vi "EmergencyStopAll.vi"() -> ()   [LabVIEW 2010]
uses:
  GenericDriveCommand.ctl
  DriveConfigGlobal.vi
panel:
  in  "stop":bool
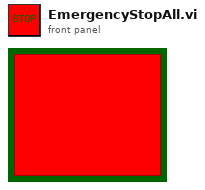
[diagram p1: front panel]
types:
  T1 = typedef "GenericDriveCommand.ctl" = string
  T2 = typedef "AxisConfigCluster.ctl" = cluster{"Channel Properties":T3, "Static Drive Configuration":T4}
  T3 = typedef "DriveProperties.ctl" = cluster{"Channel Name":string, "Vel. Default":dbl, "Acc. Default":dbl, "Vel. Max":dbl, "Vel. Min":dbl, "Acc. Max":dbl, "Acc. Min":dbl, "Pulses/unit":dbl, "Address":u8, "Pulse Offset":i32, "Pos Tolerance":dbl, "Pulses/rev":dbl, "Backlash/Eng units":dbl, "Current Pos":dbl, "Ch Status":enum16{"Active", "Offline", "Simulate"}, "Port Name":string, "Axis Transform mode":string, "Metadata Ch Name":string, "Type":string}
  T4 = typedef "DriveStaticConfig.ctl" = cluster{"Correction Gain % (CG)":u16, "Dead Band (DB)":i32, "Dead Band Window (DW)":i32, "Encoder Resolution (ER)":i32, "Step Mode  (FSB)":u16, "Position Maintenance (FSC)":u16, "Stop on Stall (FSD)":u16, "Activate OP1 on stall (FSE)":u16, "Stop on Trigger 3 (FSF)":u16, "OP2 in Deadband (FSG)":u16, "Stall Detect (FSH)":u16, "Limit Disable (LD)":u16, "Motor Resolution (MR)":enum16{"200", "400", "1000", "2000", "4000", "5000", "10000", "12800", "18000", "20000", "21600", "25000", "25400", "25600", "36000", "50000", "278528", "425984", "507904", "614400", "655360", "819200", "1024000"}, "Limit Switch Sense (OSA)":u16, "Home Position (OSB)":u16, "Home Switch Sense (OSC)":u16, "Encoder Z for Home (OSD)":u16, "Reference edge of Home (OSH)":u16, "RS232 Echo Control (SSA)":u16, "Buffer at Limit (SSG)":u16, "Buffer at Stop (SSH)":u16, "Indexer Mode  (FSA)":u16, "Type":string, "ConfigString":string, "De Power Motor":enum16{"TRUE", "FALSE"}}
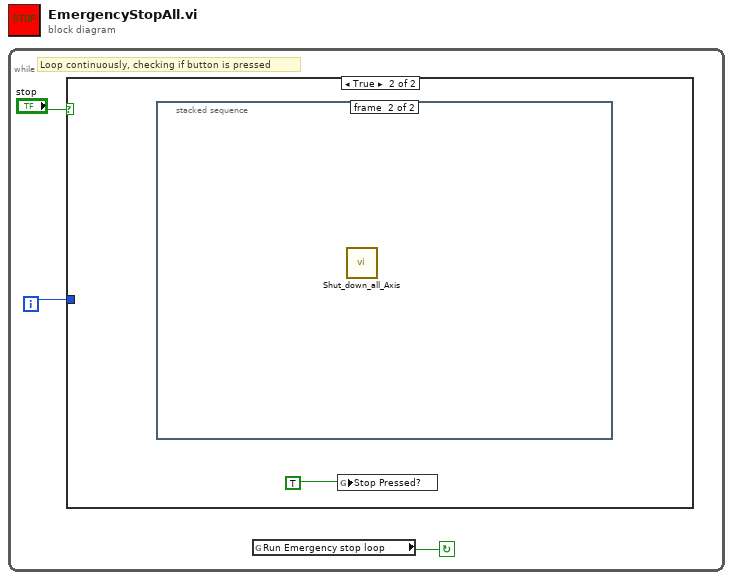
[diagram p0: block diagram]
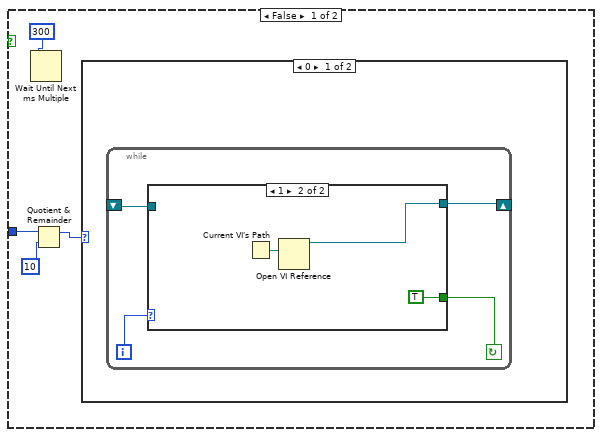
[diagram p2: hidden frame]
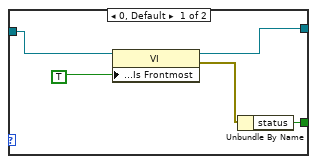
[diagram p3: hidden frame]
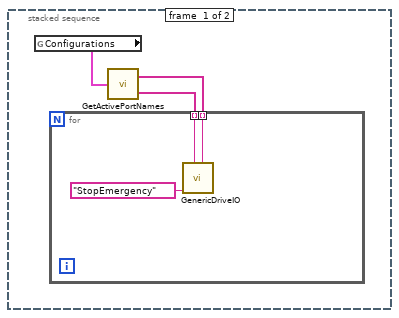
[diagram p5: hidden frame]
diagram:
  n1 = while {
    i -> [w1]
    stop <- w2 continue-if-true
    # "Loop continuously, checking if button is pressed"
    n2 = case shown="True" "stop" {
      tunnel: w1 -> [w6 _]
      frame False {
        n3 = Wait Until Next ms Multiple(millisecond multiple=300) -> ()  [unwired: 1 out]
        n4 = Quotient & Remainder(x=w6, y=10) -> (x-y*floor(x/y)=w4:i32)  [unwired: 1 out]
        n5 = case shown="0" w4 {
          frame 0 {
            n6 = while {
              shift-left: _ -> [w11]
              shift-right: [w8] -> _
              i -> [w10]
              stop <- w9 continue-if-true
              n7 = case shown="1" w10 {
                tunnel: w11 -> [w15 _]
                tunnel: [w13 TRUE ("status")] -> w9
                tunnel: [w12 w18] -> w8
                frame 0, Default {
                  n8 = property class="VI"(reference=w15, "Front Panel Window:Is Frontmost"=TRUE) -> (reference out=w12:refnum<vi>, error out=w14:errorcluster)  [unwired: 1 in]
                  n9 = Unbundle By Name(w14) -> ("status"=w13:bool)
                }
                frame 1 {
                  n10 = Current VI's Path() -> (path=w19:path)
                  n11 = Open VI Reference(vi path=w19) -> (vi reference=w18:refnum<vi>)  [unwired: 5 in, 1 out]
                }
              }
            }
          }
          frame 1, Default {
          }
        }
      }
      frame True {
        n12 = stacked-sequence {
          frame #0 {
            n13 = global read "DriveConfigGlobal.vi" "Configurations"() -> (w23:T2[])
            n14 = call "GetActivePortNames.vi"("Matched Configurations In"=w23) -> ("Port Name Array"=w22:string[], "Drive Type Array"=w21:string[])
            n15 = for {
              tunnel: w22 -> [w26] mode=indexing
              tunnel: w21 -> [w24] mode=indexing
              n16 = call "GenericDriveIO.vi"("GenericDriveCommand"=T1 "StopEmergency", "Type"=w24, "Port Name"=w26) -> ()  [unwired: 7 in, 2 out]
            }
          }
          frame #1 {
            n17 = call "Shut_down_all_Axis.vi"() -> ()  [unwired: 1 in]
          }
        }
        n18 = global write "DriveConfigGlobal.vi" "Stop Pressed?"(TRUE) -> ()
      }
    }
    n19 = global read "DriveConfigGlobal.vi" "Run Emergency stop loop"() -> (w2:bool)
  }
